vi "Is DQMH Request.vi"(8 "error in (no error)":errorcluster, 11 "VI in":refnum<vi>) -> (0 "error out":errorcluster, 2 "Is a DQMH Request":bool, 3 "VI out":refnum<vi>)   [LabVIEW 2017, in "Open DQMH Request Message Diagram.lvlib"]
doc: "Checks if the SubVI is a DQMH Request or a Request and Wait for Reply."
uses:
  Open DQMH Request Message Diagram.lvlib
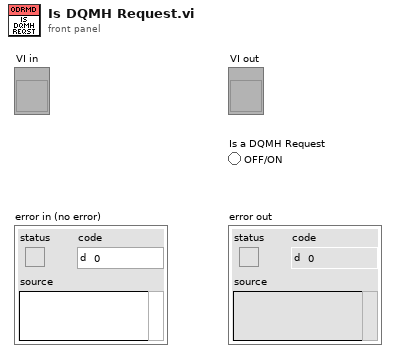
[diagram p1: front panel]
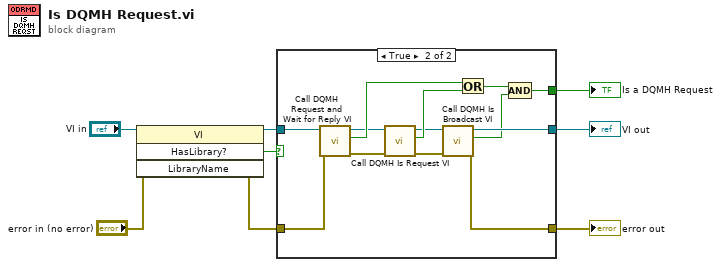
[diagram p0: block diagram]
diagram:
  n1 = invoke class="VI" method="HasLibrary?"(reference="VI in", error in="error in (no error)") -> (reference out=w5:refnum<vi>, error out=w3:errorcluster, "Has Library?"=w4:bool)  [unwired: 2 in, 1 out]
  n2 = case shown="True" w4 {
    tunnel: w5 -> [w9 w21]
    tunnel: w3 -> [w10 w20]
    tunnel: [w10 w13] -> w8
    tunnel: [w9 w12] -> w6
    tunnel: [_ w22] -> w2
    frame False {
    }
    frame True {
      n3 = call "Call DQMH Request and Wait for Reply VI.vi"("error in (no error)"=w20, "Request VI in"=w21) -> ("error out"=w16:errorcluster, "Is Request and Wait for Reply"=w19:bool, "Request VI out"=w18:refnum<vi>)  [unwired: 7 in]
      n4 = call "Call DQMH Is Request VI.vi"("error in (no error)"=w16, "Request VI in"=w18) -> ("error out"=w14:errorcluster, "Is Request"=w17:bool, "Request VI out"=w15:refnum<vi>)  [unwired: 7 in]
      n5 = call "Call DQMH Is Broadcast VI.vi"("error in (no error)"=w14, "Request VI in"=w15) -> ("error out"=w13:errorcluster, "Is Broadcast"=w11:bool, "Request VI out"=w12:refnum<vi>)  [unwired: 7 in]
      n6 = Or(x=w19, y=w17) -> (x .or. y?=w23:bool)
      n7 = Compound Arithmetic op=AND(w23, w11) -> (w22:bool)
    }
  }
  "Is a DQMH Request" <- w2
  "error out" <- w8
  "VI out" <- w6
